vi "TEST_ASIC_SUMandADDS_NEW.vi"(7 "Serial Number":string="testFile", 8 "error in (no error)":errorcluster, 11 "Instrument VISA in":T1={"AWG VISA"="AgilentGenerator1", "Oscilloscope  VISA "="AgilentOsciloscope", "Integration Board IP"="172.16.17.47", "connection ID"=refnum, "report out"=refnum, "report file path"=path "C:/Users/omartinez/Desktop/L0nL1_Results"}) -> (0 "error out":errorcluster, 3 "Instrument VISA out":T1={"AWG VISA"="AgilentGenerator1", "Oscilloscope  VISA "="AgilentOsciloscope", "Integration Board IP"="172.16.17.47", "connection ID"=refnum, "report out"=refnum, "report file path"=path "C:/Users/omartinez/Desktop/L0nL1_Results/SN_071_SumnAdds_Test.lvm"})   [LabVIEW 2012]
uses:
  <vilib>/Utility/NIReport.llb/NI_report.lvclass
  <vilib>/Utility/NIReport.llb/HTML/NI_HTML.lvclass
  <instrlib>/Agilent 8000 Series/Public/Configure/Configure Math (Binary Operation).vi
  Sum_Abrilader/L0_Sum_Adder Folder/C/Program Files/National Instruments/LabVIEW 2012/instr.lib/Agilent 8000 Series/Public/Data/Low Level/Fetch Measurement (More).vi
  <instrlib>/Agilent 8000 Series/Agilent 8000 Series.lvlib
  Sum_Abrilader/L0_Sum_Adder Folder/C/Program Files/National Instruments/LabVIEW 2012/instr.lib/Agilent 81150/Agilent 81150.lvlib
panel:
  in  "Channels \nCombinations":i32[](array[numeric])=[3, 12, 48, 96, 7, 28, 112, 15, 120, 31, 124, 63, 126, 127]
  in  "Voltages":dbl[](array[numeric])=[0.05, 0.2]
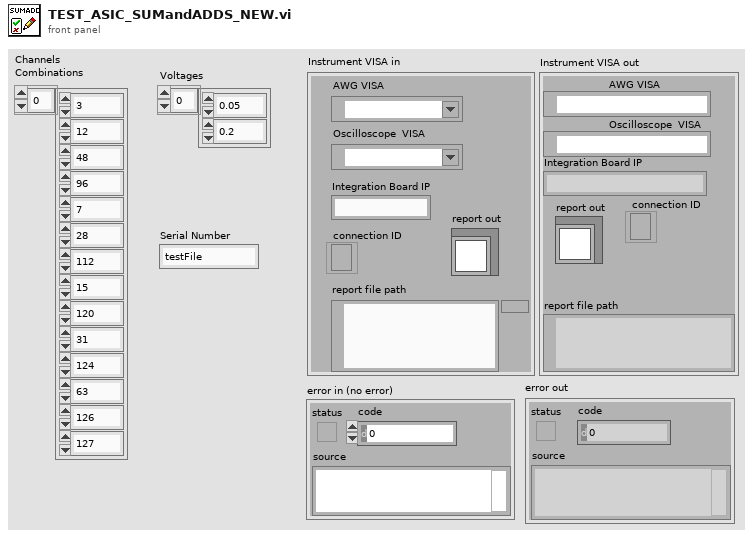
[diagram p1: front panel]
types:
  T1 = cluster{"AWG VISA":refnum<visa-resource-name>, "Oscilloscope  VISA ":refnum<visa-resource-name>, "Integration Board IP":string, "connection ID":refnum<k5>, "report out":refnum<class "NI_report.lvclass">, "report file path":path}
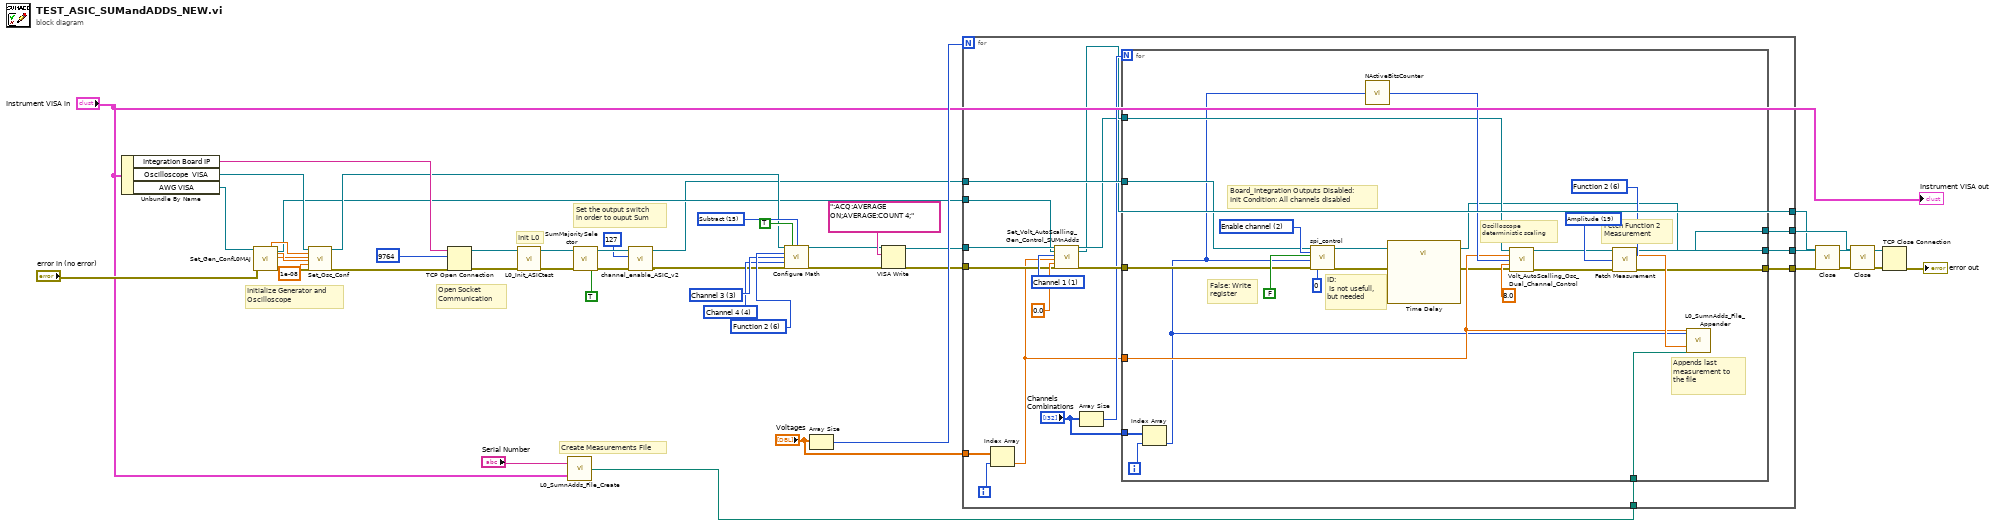
[diagram p0: block diagram]
diagram:
  w27 = u16 6 items=["Function 1"=5, "Function 2"=6, "Function 3"=7, "Function 4"=8] ("Math Channel (5: Function 1)")
  w28 = u16 15 items=["Add"=12, "Divide"=13, "Multiply"=14, "Subtract"=15, "Common Mode"=16, "Versus"=17] ("Math Operation (12: Add)")
  w26 = 3 items=["Channel 1"=1, "Channel 2"=2, "Channel 3"=3, "Channel 4"=4] ("Channel (1: Channel 1)")
  w25 = 4 items=["Channel 1"=1, "Channel 2"=2, "Channel 3"=3, "Channel 4"=4] ("Channel (1: Channel 1)")
  # "Create Measurements File"
  # "Initialize Generator and \nOscilloscope"
  # "Init L0"
  # "Set the output switch\nin order to ouput Sum"
  # "Open Socket\nCommunication"
  n1 = Unbundle By Name("Instrument VISA in") -> ("Integration Board IP"=w43:string, "Oscilloscope  VISA"=w30:refnum<visa-resource-name>, "AWG VISA"=w31:refnum<visa-resource-name>)
  n2 = call "Set_Gen_ConfL0MAJ.vi"("AWG VISA"=w31, "error in (no error)"="error in (no error)") -> ("Amplitude 1 OUT"=w37:dbl, "VISA resource name out"=w21:refnum<visa-resource-name>, "Pulse Width in seconds 1 OUT"=w36:dbl, "Trigger Level 1"=w35:dbl, "error out"=w38:errorcluster)  [unwired: 10 in, 3 out]
  n3 = call "Set_Osc_Conf.vi"("VISA resource name"=w30, "Amplitude IN"=w37, "Trigger Level IN"=w35, "Pulse Width in seconds IN"=w36, "Position 1"=1e-08, "error in (no error)"=w38) -> ("VISA resource name out"=w24:refnum<visa-resource-name>, "error out"=w32:errorcluster)  [unwired: 12 in]
  n4 = TCP Open Connection(address=w43, remote port or service name=u16 9764, error in (no error)=w32) -> (connection ID=w42:refnum<k5>, error out=w41:errorcluster)  [unwired: 2 in]
  n5 = call "L0_Init_ASICtest.vi"("error in"=w41, "connection ID in"=w42) -> ("error out"=w39:errorcluster, "connection ID out"=w40:refnum<k5>)  [unwired: 8 in]
  n6 = call "L0_SumnAdds_File_Create.vi"("input cluster"="Instrument VISA in", "Serial Number"="Serial Number") -> ("appended path"=w16:path)
  n7 = call "SumMajoritySelector.vi"("On Sum\nOff Majority"=TRUE ("On Sum\nOff Majority"), "error in (no error)"=w39, "connection ID"=w40) -> ("error out"=w15:errorcluster, "connection ID out"=w13:refnum<k5>)  [unwired: 5 in]
  n8 = call "channel_enable_ASIC_v2.vi"("error in"=w15, "Channel Combination"=u32 127, "Connection ID in"=w13) -> ("error out"=w14:errorcluster, "Connection ID out"=w12:refnum<k5>)  [unwired: 7 in]
  n9 = call-poly <instrlib>:"Configure Math.vi"("VISA resource name"=w24, "Enable Math Channel (T:Enable)"=TRUE, "Math Operation (12: Add)"=w28, "Math Channel (5: Function 1)"=w27, "Math Operand (1: Channel 1)"=w26, "Math Operand (2: Channel 2)"=w25, "error in (no error)"=w14) -> ("VISA resource name out"=w7:refnum<visa-resource-name>, "error out"=w9:errorcluster)  [unwired: 7 in]
  n10 = Array Size(array="Voltages") -> (size(s)=w22:i32)
  n11 = VISA Write(VISA resource name=w7, write buffer=":ACQ:AVERAGE ON;AVERAGE:COUNT 4;", error in (no error)=w9) -> (VISA resource name out=w6:refnum<visa-resource-name>, error out=w8:errorcluster)  [unwired: 1 out]
  n12 = for {
    N: w22 -> [_]
    tunnel: w12 -> [w62]
    tunnel: w8 -> [w57]
    tunnel: [w63] -> w4
    tunnel: "Voltages" -> [w60]
    tunnel: w6 -> [w56]
    tunnel: w21 -> [w55]
    tunnel: [w51] -> w19
    tunnel: w16 -> [w48]
    tunnel: [w47] -> w2
    tunnel: [w46] -> w1
    i -> [w61]
    w59 = 1 items=["Channel 1"=1, "Channel 2"=2, "Channel 3"=3, "Channel 4"=4] ("Channel")
    n13 = Index Array(array=w60, index=w61) -> (element=w49:dbl)
    n14 = call "Set_Volt_AutoScalling_Gen_Control_SUMnAdds.vi"("VISA Oscilloscope"=w56, "VISA Generator"=w55, "Channel"=w59, "Amplitude"=w49, "DC Offset"=0.0, "error in (no error)"=w57) -> ("VISA Oscilloscope"=w50:refnum<visa-resource-name>, "VISA Generator"=w46:refnum<visa-resource-name>, "error out"=w54:errorcluster)  [unwired: 11 in]
    n15 = Array Size(array="Channels \nCombinations") -> (size(s)=w52:i32)
    n16 = for {
      N: w52 -> [_]
      tunnel: [w74] -> w63
      tunnel: w62 -> [w83]
      tunnel: w54 -> [w82]
      tunnel: "Channels \nCombinations" -> [w80]
      tunnel: [w66] -> w51
      tunnel: w50 -> [w72]
      tunnel: w49 -> [w71]
      tunnel: w48 -> [w68]
      tunnel: [w64] -> w47
      i -> [w81]
      w79 = 19 items=["Rise Time", "Fall Time", "Frequency", "Period", "Voltage RMS(AC)", "Voltage RMS(DC)", "Voltage RMS (AC,cycle)", "Voltage RMS (DC,cycle)", "Voltage Max", "Voltage Min", "Voltage Middle", "Voltage Vpp", "Voltage High", "Voltage Low", "Voltage Average", "Voltage Average (cycle)", "Width Negative", "Width Positive", "Duty Cycle Positive", "Amplitude", "Overshoot", "Preshoot", "Voltage Base", "Voltage Upper", "Time Max", "Time Min", "Color Grade Crossing", "Color Grade Eye Width", "Color Grade Eye Height", "Color Grade Eye Q-Factory", "Color Grade Eye Duty Cycle Distortion(Percent)", "Color Grade Eye Duty Cycle Distortion(Time)", "Color Grade Eye Jitter(PP)", "Color Grade Eye Width(RMS)", "Cycle-cycle Duty Jitter(Rising)", "Cycle-cycle Duty Jitter(Falling)", "Cycle-cycle Jitter(Rising)", "Cycle-cycle Jitter(Falling)", "Cycle-cycle - Width", "Cycle-cycle + Width", "Date Rate", "Unit Interval", "FFT Delta Frequency", "FFT Delta Magnitude", "FFT Frequency", "FFT Magnitude", "Slew Rate", "Area (Entire Display)", "Area(Single Cycle)", "Duty Cycle (Rising)", "Duty Cycle (Falling)"] ("Measurement Function (0: Rise Time)")
      w78 = 6 items=["Channel 1"=1, "Channel 2"=2, "Channel 3"=3, "Channel 4"=4, "Function 1"=5, "Function 2"=6, "Function 3"=7, "Function 4"=8, "Memory 1"=9, "Memory 2"=10, "Memory 3"=11, "Memory 4"=12] ("Channel (1: Channel 1)")
      w85 = u16 2 items=["Attenuation", "Clipping", "Enable channel", "Delay line", "ASIC"] ("Device")
      # "Fetch Function 2\nMeasurement"
      # "Appends last\nmeasurement to\nthe file"
      # "Oscilloscope \ndeterministic scaling"
      # "False: Write\nregister"
      # "ID:\n Is not usefull, \nbut needed"
      # "Board_Integration Outputs Disabled:\nInit Condition: All channels disabled"
      n17 = Index Array(array=w80, index=w81) -> (element=w70:i32)
      n18 = call "spi_control.vi"("connection ID"=w83, "Device"=w85, "Read/#write"=FALSE, "Data"=w70, "error in"=w82, "Id in"=0) -> ("connection ID out"=w66:refnum<k5>, "error out 2"=w67:errorcluster)  [unwired: 6 in, 6 out]
      n19 = call "NActiveBitsCounter.vi"("Input Number"=w70) -> ("N High Bits"=w73:i32)
      n20 = call "Time Delay"("error in (no error)"=w67) -> ("error out"=w65:errorcluster)  [unwired: 10 in]
      n21 = call "Volt_AutoScalling_Osc_Dual_Channel_Control.vi"("VISA Oscilloscope"=w72, "Voltage In"=w71, "N Channels"=w73, "Offset Divider"=8.0, "error in"=w65) -> ("VISA resource name out"=w76:refnum<visa-resource-name>, "error out"=w77:errorcluster)  [unwired: 9 in]
      n22 = call-poly "Fetch Measurement.vi"("VISA resource name"=w76, "Channel (1: Channel 1)"=w78, "Measurement Function (0: Rise Time)"=w79, "error in (no error)"=w77) -> ("VISA resource name out"=w64:refnum<visa-resource-name>, "Measurement"=w75:dbl, "error out"=w74:errorcluster)  [unwired: 9 in]
      n23 = call "L0_SumnAdds_File_Appender.vi"("Vin"=w71, "CH"=w70, "Vmeas"=w75, "file path (dialog if empty)"=w68) -> ()  [unwired: 24 in]
    }
  }
  n24 = call <instrlib>:"Close.vi"("error in (no error)"=w4, "VISA resource name"=w1) -> ("error out"=w5:errorcluster)  [unwired: 9 in]
  n25 = call <instrlib>:"Close.vi"("error in (no error)"=w5, "VISA resource name"=w2) -> ("error out"=w3:errorcluster)  [unwired: 9 in]
  n26 = TCP Close Connection(connection ID=w19, error in (no error)=w3) -> (error out=→"error out":errorcluster)  [unwired: 1 in, 1 out]
  "Instrument VISA out" <- "Instrument VISA in"
